vi "util-Analog-VoltageContinuousOutput.vi"(0 "Channel(s)":tag="DAQ1/ao0", 1 "Output Array":T2(array[cluster])=[{"Waveform Type"=0, "Amplitude"=1.0, "Frequency"=10.0}] {"Frequency" format="%0.2p"; "Amplitude" format="%0.2p"; "Waveform Type" items=["Sine Wave", "Triangle Wave", "Square Wave", "Sawtooth Wave"]}, 2 "Duration(s)":dbl=5.0 caption="Delay Time (s)", 4 "Sample Rate":dbl=100000.0, 5 "Stop":bool, 7 "error in":errorcluster) -> (20 "Waveform Graph":waveform(dbl)[](graph)=[{"t0"=timestamp(0 s since 1904-01-01), "dt"=0.001, "Y"=[]}], 27 "error out":errorcluster)   [LabVIEW 2020]
doc: "This example demonstrates how to continuously re-generate analog output data from a buffer in your computer's memory.\n\nRefer to your device documentation for pinouts and hardware capabilities."
uses:
  <vilib>/Utility/error.llb/DialogType.ctl
  <vilib>/DAQmx/write.llb/DAQmx Write (Analog 1D Wfm NChan NSamp).vi
  <vilib>/DAQmx/create/channels.llb/DAQmx Create Channel (AO-Voltage-Basic).vi
  <vilib>/DAQmx/configure/timing.llb/DAQmx Timing (Sample Clock).vi
  <vilib>/DAQmx/configure/trigger.llb/DAQmx Start Trigger (Digital Edge).vi
  <vilib>/DAQmx/configure/trigger.llb/DAQmx Start Trigger (Time).vi
  <vilib>/DAQmx/configure/trigger.llb/DAQmx Start Trigger (Analog Edge).vi
  <vilib>/DAQmx/miscellaneous.llb/DAQmx Fill In Error Info.vi
  <resource>/objmgr/daqmx.rc
  <vilib>/measure/NI_MABase.lvlib
panel:
  in  "Trigger Type":T1(tab)
  in  "Digital Start Trigger Edge":i32(ring)=10280 caption="Edge" items=["Rising"=10280, "Falling"=10171]
  in  "Digital Start Trigger Source":tag="/Dev1/PFI0" caption="Source"
  in  "Digital Pause Trigger Pause When":i32(ring)=10192 caption="Pause When" items=["High"=10192, "Low"=10214]
  in  "Digital Pause Trigger Source":tag="/Dev1/PFI0" caption="Source"
  in  "Analog Start Trigger Level":dbl caption="Level" format="%0.2f"
  in  "Analog Start Trigger Hysteresis":dbl caption="Hysteresis" format="%.2f"
  in  "Analog Start Trigger Slope":i32(ring)=10280 caption="Slope" items=["Rising"=10280, "Falling"=10171]
  in  "Analog Start Trigger Source":string="APFI0" caption="Source"
  in  "Analog Pause Trigger Source":string="APFI0" caption="Source"
  in  "Analog Pause Trigger Pause When":i32(ring)=10093 caption="Pause When" items=["Above Level"=10093, "Below Level"=10107]
  in  "Analog Pause Trigger Level":dbl caption="Level" format="%.2f"
  in  "When":timestamp
  in  "Select Time\nManually":bool
  in  "Number of Samples":i32=10000
  in  "Sample Clock Source":tag="OnboardClock"
  in  "Max Voltage":dbl=5.0
  in  "Min Voltage":dbl=-5.0
  out "Actual Sample Rate":dbl=1000.0 format="%0.2f"
  # "Channel Settings"
  # "Output"
  # "Timing and\nBuffer Settings"
  # "Waveform Settings"
  # "Trigger Settings"
  # "The number of elements in the waveform array must equal the number of channels in the task."
  # "To enable triggers, select a tab above, and configure the settings.\n\nNot all hardware supports all trigger types. Refer to your device documentation for more information."
  # "This trigger type is not supported in output tasks. \n\nRefer to your device documentation for more information on which triggers are supported."
  # "This trigger type is not supported in output tasks. \n\nRefer to your device documentation for more information on which triggers are supported."
  # "If time is not manually set, task will begin after 10 seconds"
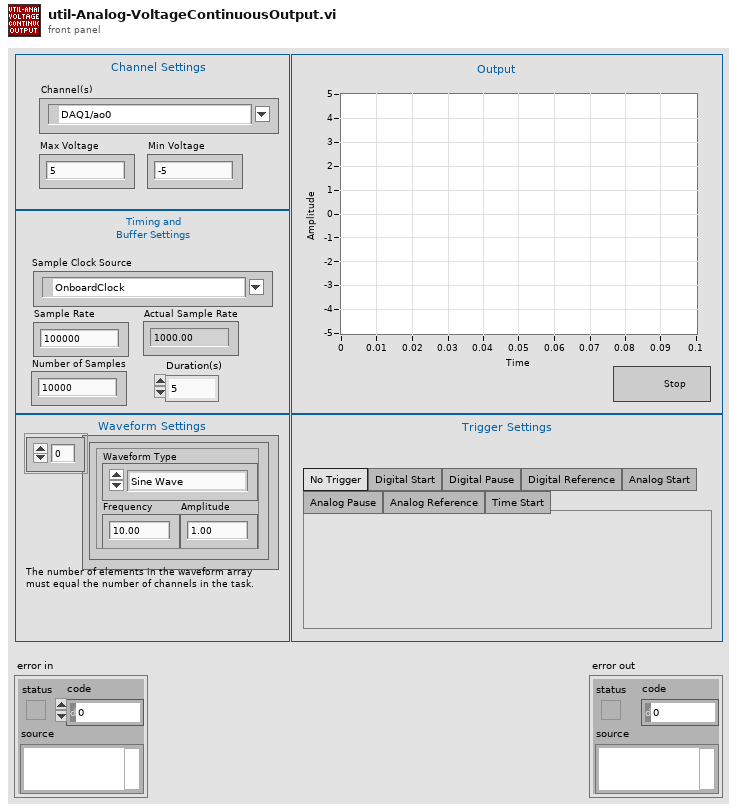
[diagram p1: front panel]
types:
  T1 = enum32{"No Trigger", "Digital Start", "Digital Pause", "Digital Reference", "Analog Start", "Analog Pause", "Analog Reference", "Time Start"}
  T2 = cluster{"Waveform Type":u16, "Amplitude":dbl, "Frequency":dbl}[]
  T3 = typedef "DialogType.ctl" = u16
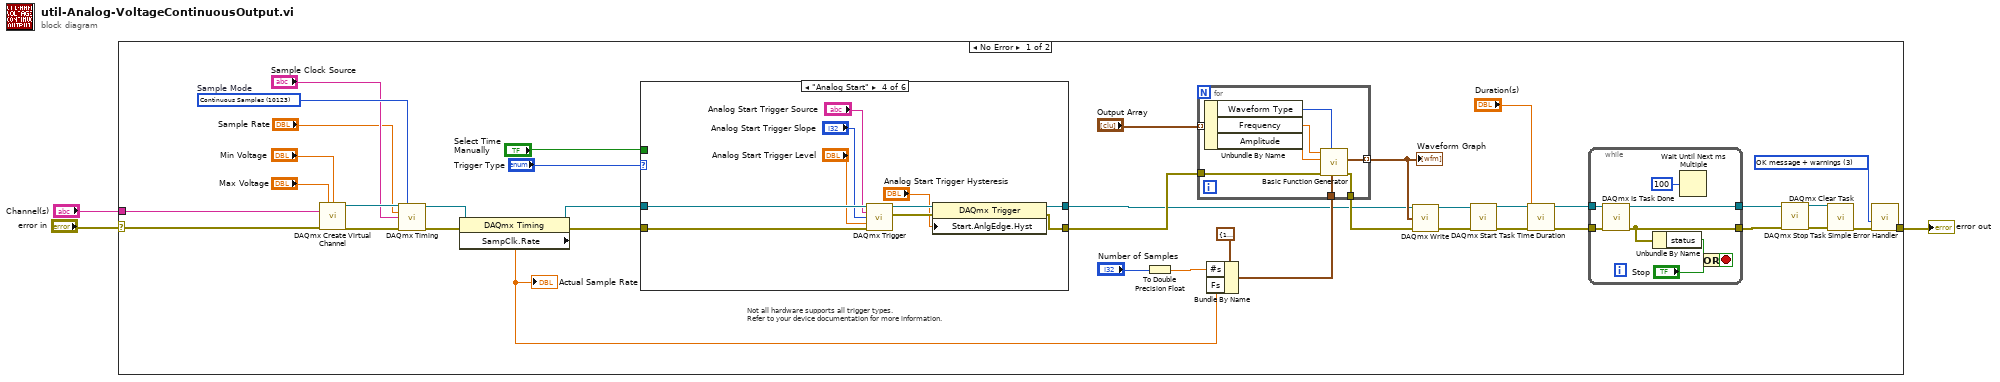
[diagram p0: block diagram]
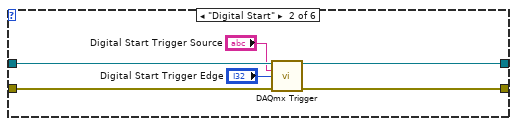
[diagram p3: hidden frame]
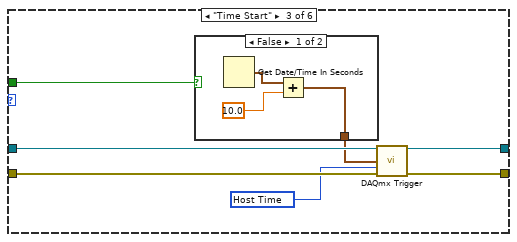
[diagram p4: hidden frame]
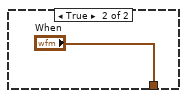
[diagram p5: hidden frame]
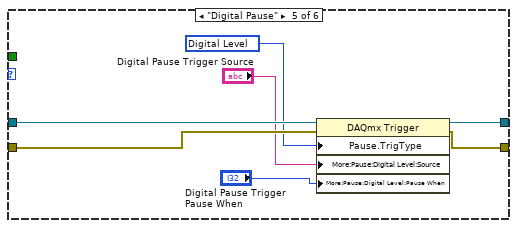
[diagram p6: hidden frame]
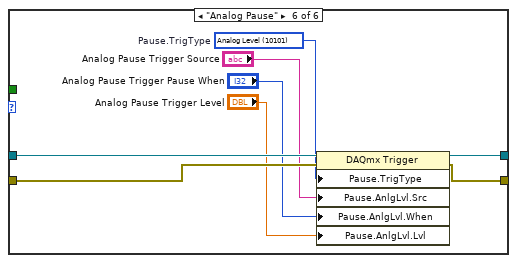
[diagram p7: hidden frame]
diagram:
  n1 = case shown="No Error" "error in" {
    selector: "error in" -> [w8 w102]
    tunnel: [w10 w102] -> w3
    tunnel: "Channel(s)" -> [w9 _]
    frame No Error {
      w16 = T3 3 items=["no dialog", "OK message", "continue or stop message", "OK message + warnings", "continue/stop + warnings"] ("type of dialog (OK msg:1)")
      w39 = 10123 items=["Finite Samples"=10178, "Continuous Samples"=10123, "Hardware Timed Single Point"=12522]  # Sample Mode
      # "Not all hardware supports all trigger types.\nRefer to your device documentation for more information."
      n2 = call-poly <vilib>:"DAQmx Create Virtual Channel.vi"("maximum value"="Max Voltage", "minimum value"="Min Voltage", "physical channels"=w9, "error in"=w8) -> ("task out"=w37:refnum<k21>, "error out"=w38:errorcluster)  [unwired: 10 in]
      n3 = call-poly <vilib>:"DAQmx Timing.vi"("task/channels in"=w37, "sample mode"=w39, "rate"="Sample Rate", "source"="Sample Clock Source", "error in"=w38) -> ("task out"=w41:refnum<k21>, "error out"=w40:errorcluster)  [unwired: 9 in]
      n4 = property class="DAQmx Timing"(reference=w41, error in=w40) -> (reference out=w14:refnum<k21>, error out=w13:errorcluster, "SampClk.Rate"=w29:dbl)
      "Actual Sample Rate" <- w29
      n5 = case shown="\"Analog Start\"" "Trigger Type" {
        tunnel: w14 -> [w43 w49 w56 w70 w77 w85]
        tunnel: w13 -> [w42 w48 w55 w69 w74 w82]
        tunnel: [w43 w47 w54 w67 w76 w84] -> w11
        tunnel: [w42 w46 w53 w66 w75 w83] -> w12
        tunnel: "Select Time\nManually" -> [_ _ w50 _ _ _]
        frame "No Trigger", Default {
        }
        frame "Digital Start" {
          n6 = call-poly <vilib>:"DAQmx Trigger.vi"("task/channels in"=w49, "source"="Digital Start Trigger Source", "edge"="Digital Start Trigger Edge", "error in"=w48) -> ("task out"=w47:refnum<k21>, "error out"=w46:errorcluster)  [unwired: 10 in]
        }
        frame "Time Start" {
          w52 = 16126 items=["Host Time"=16126, "I/O Device Time"=16127] ("timescale")
          n7 = case shown="False" w50 {
            tunnel: [w58 "When"] -> w51
            frame False {
              n8 = Get Date/Time In Seconds() -> (seconds since 1Jan1904=w59:timestamp)
              n9 = Add(x=w59, y=10.0) -> (x+y=w58:timestamp)
            }
            frame True {
            }
          }
          n10 = call-poly <vilib>:"DAQmx Trigger.vi"("task/channels in"=w56, "when"=w51, "timescale"=w52, "error in"=w55) -> ("task out"=w54:refnum<k21>, "error out"=w53:errorcluster)  [unwired: 10 in]
        }
        frame "Analog Start" {
          n11 = call-poly <vilib>:"DAQmx Trigger.vi"("task/channels in"=w70, "source"="Analog Start Trigger Source", "slope"="Analog Start Trigger Slope", "level"="Analog Start Trigger Level", "error in"=w69) -> ("task out"=w65:refnum<k21>, "error out"=w64:errorcluster)  [unwired: 9 in]
          n12 = property class="DAQmx Trigger"(reference=w65, error in=w64, "Start.AnlgEdge.Hyst"="Analog Start Trigger Hysteresis") -> (reference out=w67:refnum<k21>, error out=w66:errorcluster)
        }
        frame "Digital Pause" {
          w73 = 10152 items=["Analog Level"=10101, "Analog Window"=10103, "Digital Level"=10152, "Digital Pattern"=10398, "None"=10230] ("Pause.TrigType")
          n13 = property class="DAQmx Trigger"(reference=w77, error in=w74, "Pause.TrigType"=w73, "More:Pause:Digital Level:Source"="Digital Pause Trigger Source", "More:Pause:Digital Level:Pause When"="Digital Pause Trigger Pause When") -> (reference out=w76:refnum<k21>, error out=w75:errorcluster)
        }
        frame "Analog Pause" {
          w81 = 10101 items=["Analog Level"=10101, "Analog Window"=10103, "Digital Level"=10152, "Digital Pattern"=10398, "None"=10230]  # Pause.TrigType
          n14 = property class="DAQmx Trigger"(reference=w85, error in=w82, "Pause.TrigType"=w81, "Pause.AnlgLvl.Src"="Analog Pause Trigger Source", "Pause.AnlgLvl.When"="Analog Pause Trigger Pause When", "Pause.AnlgLvl.Lvl"="Analog Pause Trigger Level") -> (reference out=w84:refnum<k21>, error out=w83:errorcluster)
        }
      }
      n15 = To Double Precision Float(number="Number of Samples") -> (double precision float=w22:dbl)
      n16 = Bundle By Name(cluster=cluster{"Fs":dbl, "#s":dbl} {"Fs"=1000.0, "#s"=1000.0} ("sampling info"), "#s"=w22, "Fs"=w29) -> (w28:cluster{"Fs":dbl, "#s":dbl})
      n17 = for {
        tunnel: w12 -> [w93]
        tunnel: w28 -> [w92]
        tunnel: [w91] -> w25
        tunnel: "Output Array" -> [w90] mode=indexing
        tunnel: [w86] -> w23 mode=indexing
        n18 = Unbundle By Name(w90) -> ("Waveform Type"=w89:u16, "Frequency"=w88:dbl, "Amplitude"=w87:dbl)
        n19 = call <vilib>:"Basic Function Generator.vi"("sampling info"=w92, "signal type"=w89, "error in (no error)"=w93, "amplitude"=w87, "frequency"=w88) -> ("error out"=w91:errorcluster, "signal out"=w86:waveform(dbl))  [unwired: 4 in, 1 out]
      }
      "Waveform Graph" <- w23
      n20 = call-poly <vilib>:"DAQmx Write.vi"("task/channels in"=w11, "data"=w23, "error in"=w25) -> ("task out"=w27:refnum<k21>, "error out"=w26:errorcluster)  [unwired: 10 in, 1 out]
      n21 = call <vilib>:"DAQmx Start Task.vi"("task/channels in"=w27, "error in"=w26) -> ("task out"=w36:refnum<k21>, "error out"=w6:errorcluster)  [unwired: 12 in]
      n22 = call "Time Duration"("error in (no error)"=w6, "Delay Time (s)"="Duration(s)") -> ("error out"=w5:errorcluster)  [unwired: 9 in]
      n23 = while {
        tunnel: w36 -> [w101]
        tunnel: w5 -> [w100]
        tunnel: [w97] -> w17
        tunnel: [w98] -> w18
        stop <- w99 stop-if-true
        n24 = call <vilib>:"DAQmx Is Task Done.vi"("task/channels in"=w101, "error in"=w100) -> ("task out"=w98:refnum<k21>, "error out"=w97:errorcluster)  [unwired: 11 in, 1 out]
        n25 = Unbundle By Name(w97) -> ("status"=w96:bool)
        n26 = Wait Until Next ms Multiple(millisecond multiple=u32 100) -> ()  [unwired: 1 out]
        n27 = Or(x=w96, y="Stop") -> (x .or. y?=w99:bool)
      }
      n28 = call <vilib>:"DAQmx Stop Task.vi"("task/channels in"=w18, "error in"=w17) -> ("task out"=w20:refnum<k21>, "error out"=w19:errorcluster)  [unwired: 12 in]
      n29 = call <vilib>:"DAQmx Clear Task.vi"("task in"=w20, "error in"=w19) -> ("error out"=w35:errorcluster)  [unwired: 13 in]
      n30 = call <vilib>:"Simple Error Handler.vi"("type of dialog (OK msg:1)"=w16, "error in (no error)"=w35) -> ("error out"=w10:errorcluster)  [unwired: 3 in, 4 out]
    }
    frame Error {
    }
  }
  "error out" <- w3
